vi "Get Serial Number.vi"(8 "error in":errorcluster, 11 "Alicat Device in":refnum<class "Alicat Device.lvclass">=refnum) -> (0 "error out":errorcluster, 2 "Serial Number":string, 3 "Alicat Device out":refnum<class "Alicat Device.lvclass">)   [LabVIEW 2014]
uses:
  reusable/Session APIs/Serial/Serial Session.lvclass
  reusable/Session APIs/Serial/Public/Get Data/Get String.vi
  Alicat Device.lvclass
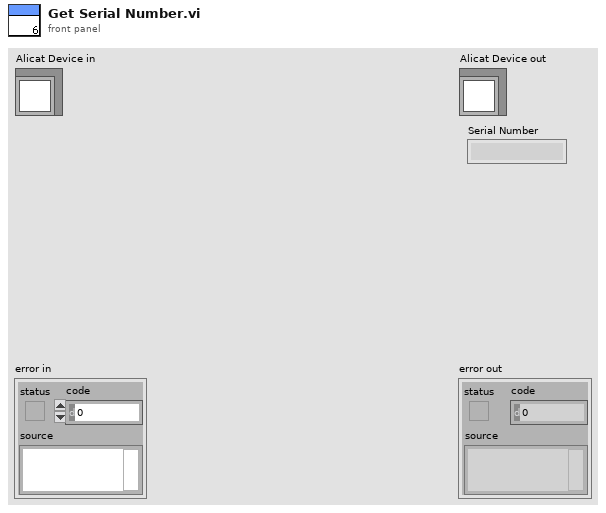
[diagram p1: front panel]
types:
  T1 = typedef "Serial Session.lvclass/Session Handle.ctl" = refnum<data-value>
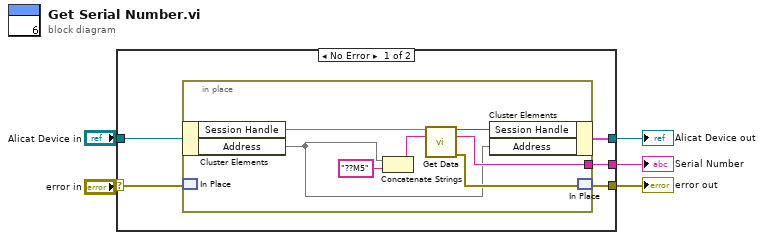
[diagram p0: block diagram]
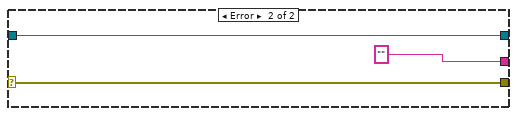
[diagram p2: hidden frame]
diagram:
  n1 = case shown="No Error" "error in" {
    selector: "error in" -> [w9 w20]
    tunnel: "Alicat Device in" -> [w10 w19]
    tunnel: [w7 w20] -> w1
    tunnel: [w8 w19] -> w3
    tunnel: [w6 "" ("DataOut")] -> w4
    frame No Error {
      n2 = in-place {
        in-place-border: [w15] -> w6
        n3 = in-place-cluster #1(w10) -> ("Session Handle"=w14, "Address"=w13)
        n4 = in-place-match #2(w9) -> ()  [unwired: 1 out]
        n5 = Concatenate Strings(w13, "??M5" ("string")) -> (w11:string)
        n6 = call-poly "Get Data.vi"("Session Handle in"=w14, "CMD"=w11) -> ("Session Handle out"=w17:T1, "DataOut"=w15:string, "error out"=w16:errorcluster)  [unwired: 11 in]
        n7 = in-place-cluster #1("Session Handle"=w17, "Address"=w13) -> (w8:cluster{})
        n8 = in-place-match #2(w16) -> (w7:errorcluster)
      }
    }
    frame Error {
    }
  }
  "error out" <- w1
  "Alicat Device out" <- w3
  "Serial Number" <- w4
